vi "DiffDriveKinematicsConstraint_New.vi"(9 "DIFF_DRIVE_KINEMATICS":T1 {"TrackWidth_Meters" format="%20.4f"}, 10 "Max Accel (M/S2)":dbl=999999.0 format="%20.4f", 11 "Max Speed (M/S)":dbl format="%20.4f") -> (3 "DIFF_DRIVE_KINE_CONSTRAINT":T2={"Max Speed (M/S)"=0.0, "DIFF_DRIVE_KINEMATICS"={"TrackWidth_Meters"=0.0}, "Max Accel (M/S2)"=99999.0} {"Max Accel (M/S2)" format="%20.4f"; "DIFF_DRIVE_KINEMATICS"."TrackWidth_Meters" format="%20.4f"; "Max Speed (M/S)" format="%20.4f"})   [LabVIEW 2019, in "Trajectory_Library.lvlib"]
doc: "Constructs a differential drive dynamics constraint.\n\n\nParameters:\n - MaxSpeed - Max speed (meters/sec)\n - DiffDriveKinematics - Diff Drive Kinematics data structure\n\nReturns\n - DiffDriveKineConstraint - Constraint data structure."
uses:
  Trajectory_Library.lvlib
  TypeDef/TRAJ_CONSTRAINT_DIIF_DRIVE_KINEMATICS.ctl
  TypeDef/DIFF_DRIVE_KINEMATICS.ctl
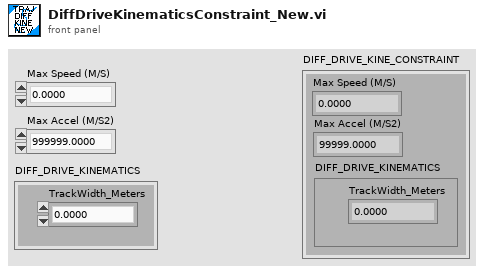
[diagram p1: front panel]
types:
  T1 = typedef "Trajectory_Library.lvlib/DIFF_DRIVE_KINEMATICS.ctl" = cluster{"TrackWidth_Meters":dbl}
  T2 = typedef "Trajectory_Library.lvlib/TRAJ_CONSTRAINT_DIIF_DRIVE_KINEMATICS.ctl" = cluster{"Max Speed (M/S)":dbl, "DIFF_DRIVE_KINEMATICS":T1, "Max Accel (M/S2)":dbl}
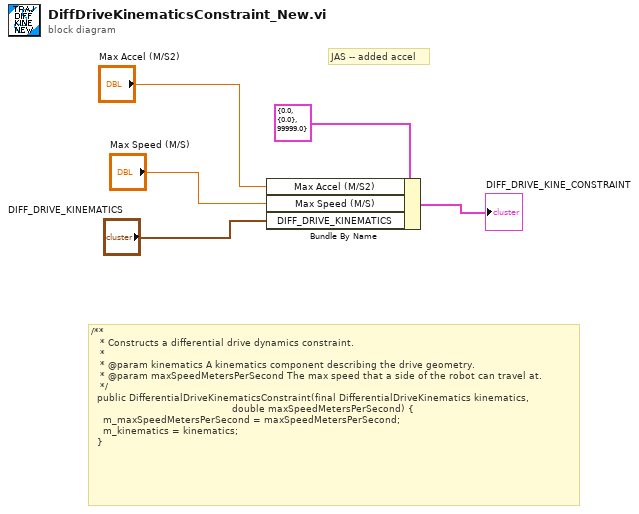
[diagram p0: block diagram]
diagram:
  # "JAS -- added accel"
  # "/**\n   * Constructs a differential drive dynamics constraint.\n   *\n   * @param kinematics A kinematics component describing the drive geometry.\n   * @param maxSpeedMetersPerSecond The max speed that a side of the robot can travel at.\n   */\n  public DifferentialDriveKinematicsConstraint(final DifferentialDriveKinematics kinematics,\n                                               double maxSpeedMetersPerSecond) {\n    m_maxSpeedMetersPerSecond = maxSpeedMetersPerSecond;\n    m_kinematics = kinematics;\n  }"
  n1 = Bundle By Name(cluster=T2 {"Max Speed (M/S)"=0.0, "DIFF_DRIVE_KINEMATICS"={"TrackWidth_Meters"=0.0}, "Max Accel (M/S2)"=99999.0} ("DIFF_DRIVE_KINE_CONSTRAINT"), "Max Accel (M/S2)"="Max Accel (M/S2)", "Max Speed (M/S)"="Max Speed (M/S)", "DIFF_DRIVE_KINEMATICS"="DIFF_DRIVE_KINEMATICS") -> (→"DIFF_DRIVE_KINE_CONSTRAINT":T2)
